vi "Towerlight GV.vi"() -> ()   [LabVIEW 2017]
uses:
  controls/Towerlight.ctl
panel:
  out "Flash Successful":bool
  in  "Flash":bool
  out "Maint DO":u32
  in  "Status":T1
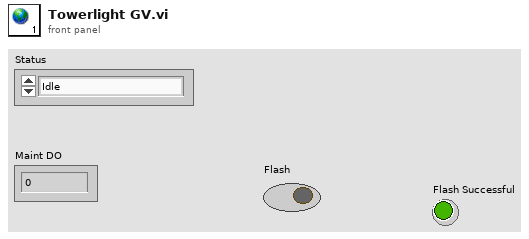
[diagram p1: front panel]
types:
  T1 = typedef "Towerlight.ctl" = enum16{"Idle", "Error", "Attention", "Running", "Maintenance", "Fail"}
diagram:
